vi "Pipe Var Intf - Wait ACK.vi"(7 "timeout [ms]":i32=3000, 8 "error in (no error)":errorcluster, 11 "pipe handle":i32) -> (0 "error out":errorcluster, 3 "pipe handle out":i32)   [LabVIEW 2020, in "GOLPI library.lvlib"]
doc: "Waits for response from Octave's golpi_pipe_receive()."
uses:
  GOLPI library.lvlib
  <vilib>/Utility/error.llb/Error Cluster From Error Code.vi
  <vilib>/ErrorRing/Error Ring.xnode
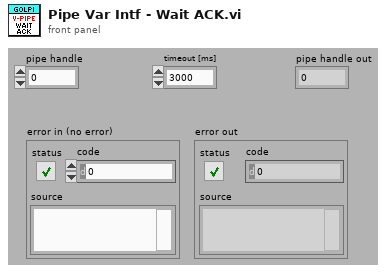
[diagram p1: front panel]
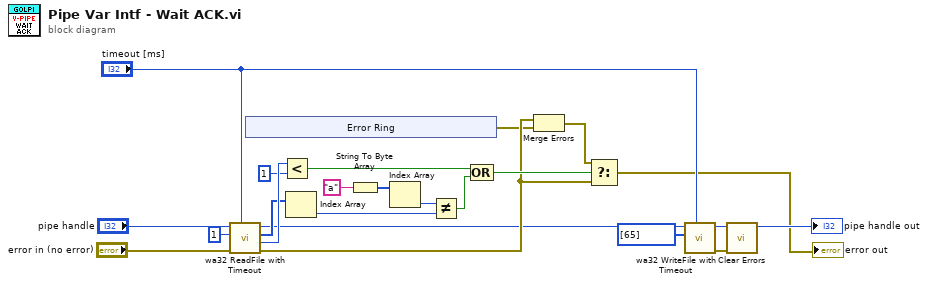
[diagram p0: block diagram]
diagram:
  n1 = call "wa32 ReadFile with Timeout.vi"("timeout [ms]"="timeout [ms]", "error in (no error)"="error in (no error)", "read count (0: all)"=1, "pipe handle"="pipe handle") -> ("error out"=w9:errorcluster, "read count"=w20:u32, "data out"=w17:u8[], "pipe handle out"=w5:i32)  [unwired: 4 in]
  n2 = xnode "Error Ring"() -> ("error out"=w8:errorcluster)
  n3 = Less?(x=w20, y=u32 1) -> (x < y?=w18:bool)
  n4 = Index Array(array=w17) -> (element=w16:u8)  [unwired: 1 in]
  n5 = String To Byte Array(string="a") -> (unsigned byte array=w13:u8[])
  n6 = Index Array(array=w13) -> (element=w12:u8)  [unwired: 1 in]
  n7 = Not Equal?(x=w12, y=w16) -> (x != y?=w15:bool)
  n8 = Compound Arithmetic op=OR(w18, w15) -> (w11:bool)
  n9 = Merge Errors(w9, w8) -> (w10:errorcluster)
  n10 = Select(t=w10, s=w11, f=w9) -> (s? t:f=→"error out":errorcluster)
  n11 = call "wa32 WriteFile with Timeout.vi"("timeout [ms]"="timeout [ms]", "data"=u8[] [65], "pipe handle"=w5) -> ("error out"=w1:errorcluster, "pipe handle out"=→"pipe handle out":i32)  [unwired: 6 in, 1 out]
  n12 = call <vilib>:"Clear Errors.vi"("error in (no error)"=w1) -> ()  [unwired: 5 in, 2 out]
